vi "ComputePiezoParameters.vi"(0 "Frame per fringe":dbl=5.0 format="%.2f", 1 "Wavelength":dbl[unit]=2.2e-06 format="%.2f", 2 "READOUT":T2, 4 "Autcollimation":bool) -> (5 "OPD stroke":dbl[unit], 6 "WAVE":T1={"Speed"=0.0, "Stiffness (0.95)"=0.95, "Linear Stroke"=0.0, "Delay"=0.0} {"Delay" format="%.2f"; "Linear Stroke" format="%.2f"; "Stiffness (0.95)" format="%.2f"; "Speed" format="%.2f"}, 7 "OPD per pixel":dbl[unit])   [LabVIEW 2009]
uses:
  Nicmos/Controls/NICMOS.READOUT.ctl
  Piezo/Controls/PIEZO.WAVE.ctl
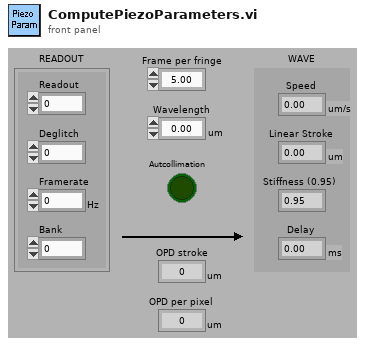
[diagram p1: front panel]
types:
  T1 = typedef "PIEZO.WAVE.ctl" = cluster{"Speed":dbl[unit], "Stiffness (0.95)":dbl, "Linear Stroke":dbl[unit], "Delay":dbl[unit]}
  T2 = typedef "NICMOS.READOUT.ctl" = cluster{"Readout":i32, "Deglitch":i32, "Framerate":dbl[unit], "Bank":i32}
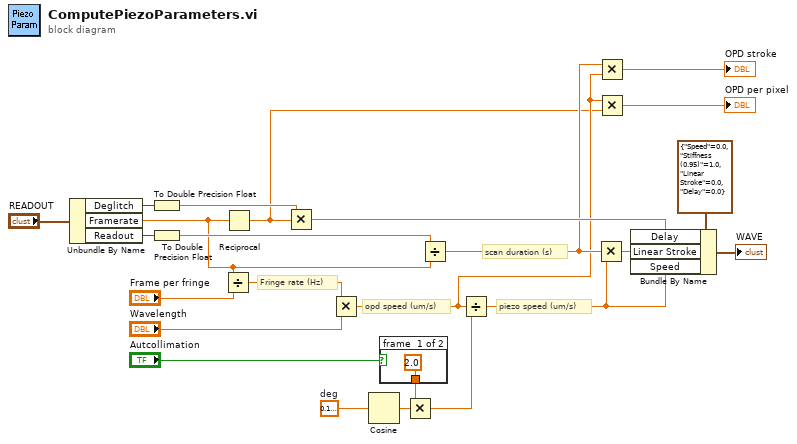
[diagram p0: block diagram]
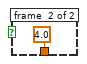
[diagram p2: hidden frame]
diagram:
  w24 = dbl[unit] 0.17453292519943295  # deg
  # "Fringe rate (Hz)"
  # "scan duration (s)"
  # "piezo speed (um/s)"
  # "opd speed (um/s)"
  n1 = Unbundle By Name("READOUT") -> ("Deglitch"=w13:i32, "Framerate"=w12:dbl[unit], "Readout"=w11:i32)
  n2 = To Double Precision Float(number=w13) -> (double precision float=w17:dbl)
  n3 = To Double Precision Float(number=w11) -> (double precision float=w19:dbl)
  n4 = Divide(x=w12, y="Frame per fringe") -> (x/y=w18:dbl[unit])
  n5 = Reciprocal(x=w12) -> (1/x=w2:dbl[unit])
  n6 = Multiply(x=w17, y=w2) -> (x*y=w7:dbl[unit])
  n7 = Multiply(x=w18, y="Wavelength") -> (x*y=w3:dbl[unit])
  n8 = Cosine(x=w24) -> (cos(x)=w22:dbl)
  n9 = case shown="False" "Autcollimation" {
    tunnel: [2.0 ("x") 4.0 ("x")] -> w21
    frame #0 {
    }
    frame #1 {
    }
  }
  n10 = Multiply(x=w22, y=w21) -> (x*y=w23:dbl)
  n11 = Divide(x=w19, y=w12) -> (x/y=w5:dbl[unit])
  n12 = Divide(x=w3, y=w23) -> (x/y=w6:dbl[unit])
  n13 = Multiply(x=w5, y=w6) -> (x*y=w8:dbl[unit])
  n14 = Multiply(x=w5, y=w3) -> (x*y=→"OPD stroke":dbl[unit])
  n15 = Multiply(x=w3, y=w2) -> (x*y=→"OPD per pixel":dbl[unit])
  n16 = Bundle By Name(cluster=T1 {"Speed"=0.0, "Stiffness (0.95)"=1.0, "Linear Stroke"=0.0, "Delay"=0.0} ("WAVE"), "Delay"=w7, "Linear Stroke"=w8, "Speed"=w6) -> (→"WAVE":T1)
